vi "Shift Logic.vi"(7 "Engine Speed (rad/s)":sgl, 9 "Down Threshold":sgl, 10 "Up Threshold":sgl, 11 "Vehicle Speed (mph)":sgl) -> (2 "Gear":sgl)   [LabVIEW 2016, in "NI-PCG Vehicle Model.lvlib"]
uses:
  NI-PCG Vehicle Model.lvlib
  Types/Gear Select State.ctl
  Globals/Parameters.vi
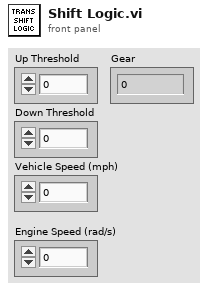
[diagram p1: front panel]
types:
  T1 = typedef "NI-PCG Vehicle Model.lvlib/Engine Parameters.ctl" = cluster{"Ambient Parameters":cluster{"Temperature (K)":sgl, "Pressure (Pa)":sgl}, "Air Parameters":cluster{"R (Ideal Gas Constant)":sgl, "Molecular Weight":sgl, "Cp (Specific Heat Constant)":sgl, "Density (kg/m^3)":sgl, "Stoichiometric A/F Ratio":sgl}, "Engine Geometry Parameters":cluster{"Cylinder Volume (l)":sgl, "J (Rotational Moment of Inertia)":sgl, "Minimuim Engine Speed":sgl, "Maximum Engine Speed":sgl, "Intake Manifold Volume (l)":sgl}, "Volumetric Efficiency Map":cluster{"MAP":sgl[], "RPM":sgl[], "Table":sgl[][]}, "Fuel LHV (J/kg)":sgl, "Combustion Efficiency Map":cluster{"Spark Timing (deg BTDC))":sgl[], "Engine Speed (RPM)":sgl[], "Combustion Efficiency":sgl[][]}, "Thermodynamic Efficiency":sgl}
  T2 = typedef "NI-PCG Vehicle Model.lvlib/Transmission Parameters.ctl" = cluster{"Final Drive Ratio":sgl, "Transmission Gear Ratios":cluster{"Gears":sgl[], "Gear Ratios":sgl[]}, "Torque Converter Map":cluster{"Speed Ratio":sgl[], "K Factor":sgl[], "Torque Ratio":sgl[]}, "Upshift Throttle":sgl[], "Downshift Throttle":sgl[], "Upshift Table":sgl[][], "Downshift Table":sgl[][], "Wait Time":u8}
  T3 = typedef "NI-PCG Vehicle Model.lvlib/Vehicle Parameters.ctl" = cluster{"Vehicle Mass (kg)":sgl, "Vehicle Cd":sgl, "Vehicle Frontal Area (m^2)":sgl, "Wheel Radius (m)":sgl, "Wheel Rolling Resistance":sgl}
  T4 = cluster{"Engine Parameters":T1, "Transmission Parameters":T2, "Vehicle Parameters":T3}
  T5 = typedef "NI-PCG Vehicle Model.lvlib/Gear Select State.ctl" = enum16{"Steady-State", "Upshifting", "Downshifting"}
  T6 = typedef "Gear Select State.ctl" = enum16{"Steady-State", "Upshifting", "Downshifting"}
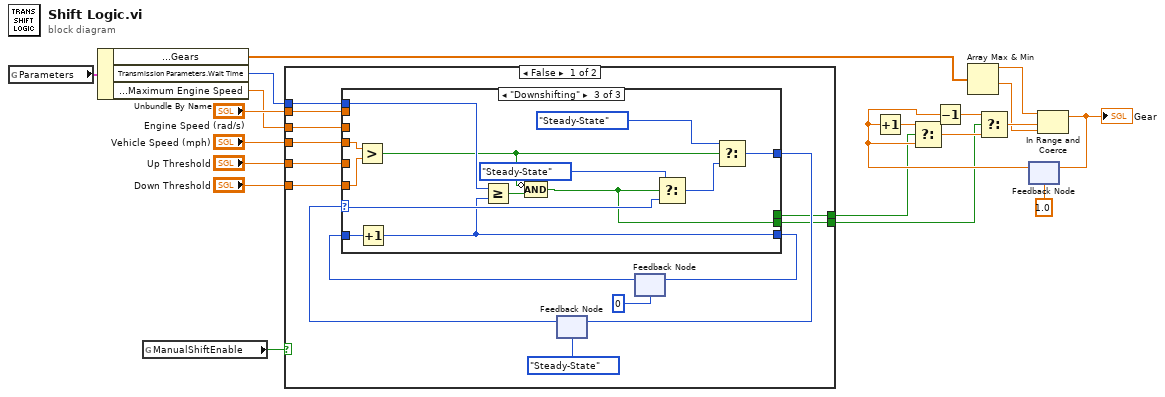
[diagram p0: block diagram]
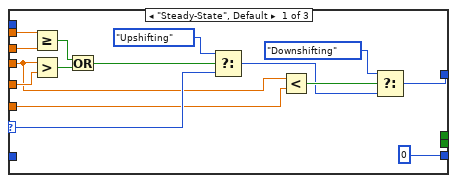
[diagram p2: hidden frame]
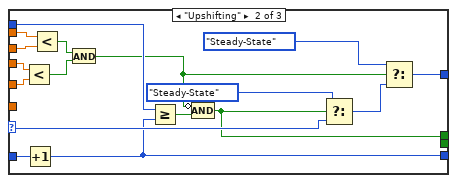
[diagram p3: hidden frame]
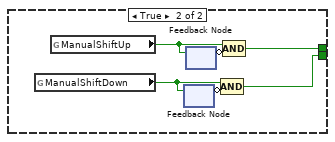
[diagram p4: hidden frame]
diagram:
  n1 = global read "Parameters.vi" "Parameters"() -> (w6:T4)
  n2 = Unbundle By Name(w6) -> ("Transmission Parameters.Transmission Gear Ratios.Gears"=w16:sgl[], "Transmission Parameters.Wait Time"=w10:u8, "Engine Parameters.Engine Geometry Parameters.Maximum Engine Speed"=w1:sgl)
  n3 = global read "Parameters.vi" "ManualShiftEnable"() -> (w3:bool)
  n4 = case shown="False" w3 {
    tunnel: w10 -> [w32 _]
    tunnel: "Vehicle Speed (mph)" -> [w31 _]
    tunnel: "Up Threshold" -> [w30 _]
    tunnel: "Down Threshold" -> [w29 _]
    tunnel: [w24 w81] -> w5
    tunnel: [w23 w80] -> w4
    tunnel: w1 -> [w21 _]
    tunnel: "Engine Speed (rad/s)" -> [w22 _]
    frame False {
      n5 = feedback #1(Gear_Select_State."Steady-State" ("Gear Selection State")) -> (w33:T6)
      n6 = feedback #2(u8 0) -> (w27:u8)
      n7 = case shown="\"Downshifting\"" w33 {
        selector: w33 -> [w48 w61 w75]
        tunnel: w32 -> [_ w66 w79]
        tunnel: w31 -> [w42 w65 w78]
        tunnel: w30 -> [w49 w64 _]
        tunnel: w29 -> [w43 _ w68]
        tunnel: [w41 w58 w72] -> w28
        tunnel: w27 -> [_ w62 w76]
        tunnel: [u8 0 w56 w69] -> w25
        tunnel: [_ w55 _] -> w24
        tunnel: [_ _ w67] -> w23
        tunnel: w22 -> [w39 w54 _]
        tunnel: w21 -> [w38 w53 _]
        frame "Steady-State", Default {
          n8 = Greater Or Equal?(x=w39, y=w38) -> (x >= y?=w37:bool)
          n9 = Greater?(x=w42, y=w49) -> (0:w36:bool)
          n10 = Or(x=w37, y=w36) -> (x .or. y?=w35:bool)
          n11 = Select(t=Gear_Select_State."Upshifting", s=w35, f=w48) -> (s? t:f=w45:T6)
          n12 = Less?(x=w42, y=w43) -> (x < y?=w46:bool)
          n13 = Select(t=Gear_Select_State."Downshifting", s=w46, f=w45) -> (s? t:f=w41:T6)
        }
        frame "Upshifting" {
          n14 = Less?(x=w65, y=w64) -> (x < y?=w51:bool)
          n15 = Increment(x=w62) -> (x+1=w56:u8)
          n16 = Less?(x=w54, y=w53) -> (x < y?=w52:bool)
          n17 = And(x=w52, y=w51) -> (x .and. y?=w50:bool)
          n18 = Greater Or Equal?(x=w66, y=w56) -> (x >= y?=w57:bool)
          n19 = Compound Arithmetic op=AND(invert w50, w57) -> (w55:bool)
          n20 = Select(t=Gear_Select_State."Steady-State", s=w55, f=w61) -> (s? t:f=w59:T6)
          n21 = Select(t=Gear_Select_State."Steady-State", s=w50, f=w59) -> (s? t:f=w58:T6)
        }
        frame "Downshifting" {
          n22 = Greater?(x=w78, y=w68) -> (0:w71:bool)
          n23 = Increment(x=w76) -> (x+1=w69:u8)
          n24 = Greater Or Equal?(x=w79, y=w69) -> (x >= y?=w70:bool)
          n25 = Compound Arithmetic op=AND(invert w71, w70) -> (w67:bool)
          n26 = Select(t=Gear_Select_State."Steady-State", s=w67, f=w75) -> (s? t:f=w73:T6)
          n27 = Select(t=Gear_Select_State."Steady-State", s=w71, f=w73) -> (s? t:f=w72:T6)
        }
      }
      n28 = feedback-in #1(w28) -> ()
      n29 = feedback-in #2(w25) -> ()
    }
    frame True {
      n30 = global read "Parameters.vi" "ManualShiftDown"() -> (w85:bool)
      n31 = global read "Parameters.vi" "ManualShiftUp"() -> (w83:bool)
      n32 = feedback #3() -> (w84:bool)  [unwired: 1 in]
      n33 = feedback-in #3(w85) -> ()
      n34 = feedback #4() -> (w82:bool)  [unwired: 1 in]
      n35 = feedback-in #4(w83) -> ()
      n36 = Compound Arithmetic op=AND(w85, invert w84) -> (w80:bool)
      n37 = Compound Arithmetic op=AND(w83, invert w82) -> (w81:bool)
    }
  }
  n38 = Array Max & Min(array=w16) -> (max value=w15:sgl, min value=w14:sgl)  [unwired: 2 out]
  n39 = feedback #5(sgl 1.0) -> (w11:sgl)
  n40 = Increment(x=w11) -> (x+1=w20:sgl)
  n41 = Select(t=w20, s=w5, f=w11) -> (s? t:f=w19:sgl)
  n42 = Decrement(x=w11) -> (x-1=w18:sgl)
  n43 = Select(t=w18, s=w4, f=w19) -> (s? t:f=w17:sgl)
  n44 = In Range and Coerce(upper limit=w15, x=w17, lower limit=w14) -> (coerced(x)=w13:sgl)  [unwired: 1 out]
  "Gear" <- w13
  n45 = feedback-in #5(w13) -> ()
